vi "WaitForConnection.vi"(8 "error in (no error)":errorcluster, 11 "TcpServer in":refnum<class "TcpServer.lvclass">) -> (0 "error out":errorcluster, 3 "TcpServer out":refnum<class "TcpServer.lvclass">)   [LabVIEW 2022 SP3, in "TcpServer.lvlib" / "TcpServer.lvclass"]
uses:
  TcpServer.lvclass
  C:/Users/jakub/repos/gh/sw4sys/lv-tcp-server-sample/LoggingActor/Source/LoggingActor/LoggingActor/LoggingActor.lvclass
  C:/Program Files (x86)/National Instruments/LabVIEW 2022/vi.lib/ActorFramework/Actor/Actor.lvclass
  TcpServer.lvclass/TcpServer.ctl
  LoggingActor/Source/LoggingActor/LoggingActor/LoggingActor.lvclass/LoggingActor.ctl
  Connection/Connection/Connection.lvclass
  TcpSocket/Source/TcpSocket/Connection/Connection.lvclass/Connection.ctl
  Connection/Connection Messages/Initialize Msg/Initialize Msg.lvclass/Initialize Msg.ctl
  <vilib>/ActorFramework/Message Enqueuer/Message Enqueuer.lvclass/Message Enqueuer.ctl
  <vilib>/ActorFramework/Actor/Actor.lvclass/Actor.ctl
  TcpSocket/Source/TcpSocket/Connection/Read Address.vi
  TcpSocket/Source/TcpSocket/Connection/Read Port.vi
  TcpSocket/Source/TcpSocket/Connection/Read Connection.vi
  TcpSocket/Source/TcpSocket/Connection/Read ReadMode.vi
  TcpSocket/Source/TcpSocket/Connection/Read ReadTimeout.vi
  TcpSocket/Source/TcpSocket/Connection/Read WriteTimeout.vi
  LoggingActor/Source/LoggingActor/LoggingActor/Read Logger.vi
  <vilib>/ActorFramework/Message Enqueuer/Enqueue.vi
  <vilib>/ActorFramework/Message Enqueuer/Init from Existing Queue.vi
  Connection/Connection Messages/Initialize Msg/Initialize Msg.lvclass
  C:/Program Files (x86)/National Instruments/LabVIEW 2022/vi.lib/ActorFramework/Message/Message.lvclass
  TcpServer Messages/WaitForConnection Msg/WaitForConnection Msg.lvclass
  <vilib>/ActorFramework/Message Priority Queue/Priority Enqueue.vi
  Logger/Source/Logger/Logger.lvclass
  <vilib>/ActorFramework/Message Enqueuer/Message Enqueuer.lvclass
  TcpSocket/Source/TcpSocket/TcpServer/TcpServer.lvclass
  <vilib>/ActorFramework/Actor/Actor.lvclass
  TcpSocket/Source/TcpSocket/Connection/Connection.lvclass
  C:/Users/jakub/repos/gh/sw4sys/lv-tcp-server-sample/TcpServerSample/Source/TcpServerSample/Connection/Connection/Connection.lvclass
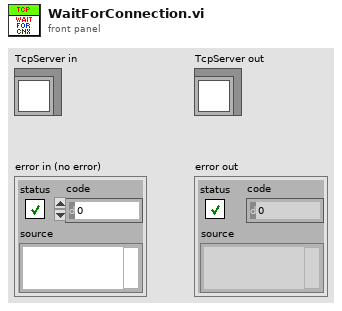
[diagram p1: front panel]
types:
  T1 = typedef "TcpServer.lvlib/TcpServer.lvclass/_ServerState.ctl" = enum16{"Idle", "Running"}
  T2 = map{u64, refnum<class "Message Enqueuer.lvclass">}
  T3 = enum16{"Standard", "Buffered", "CRLF", "Immediate"}
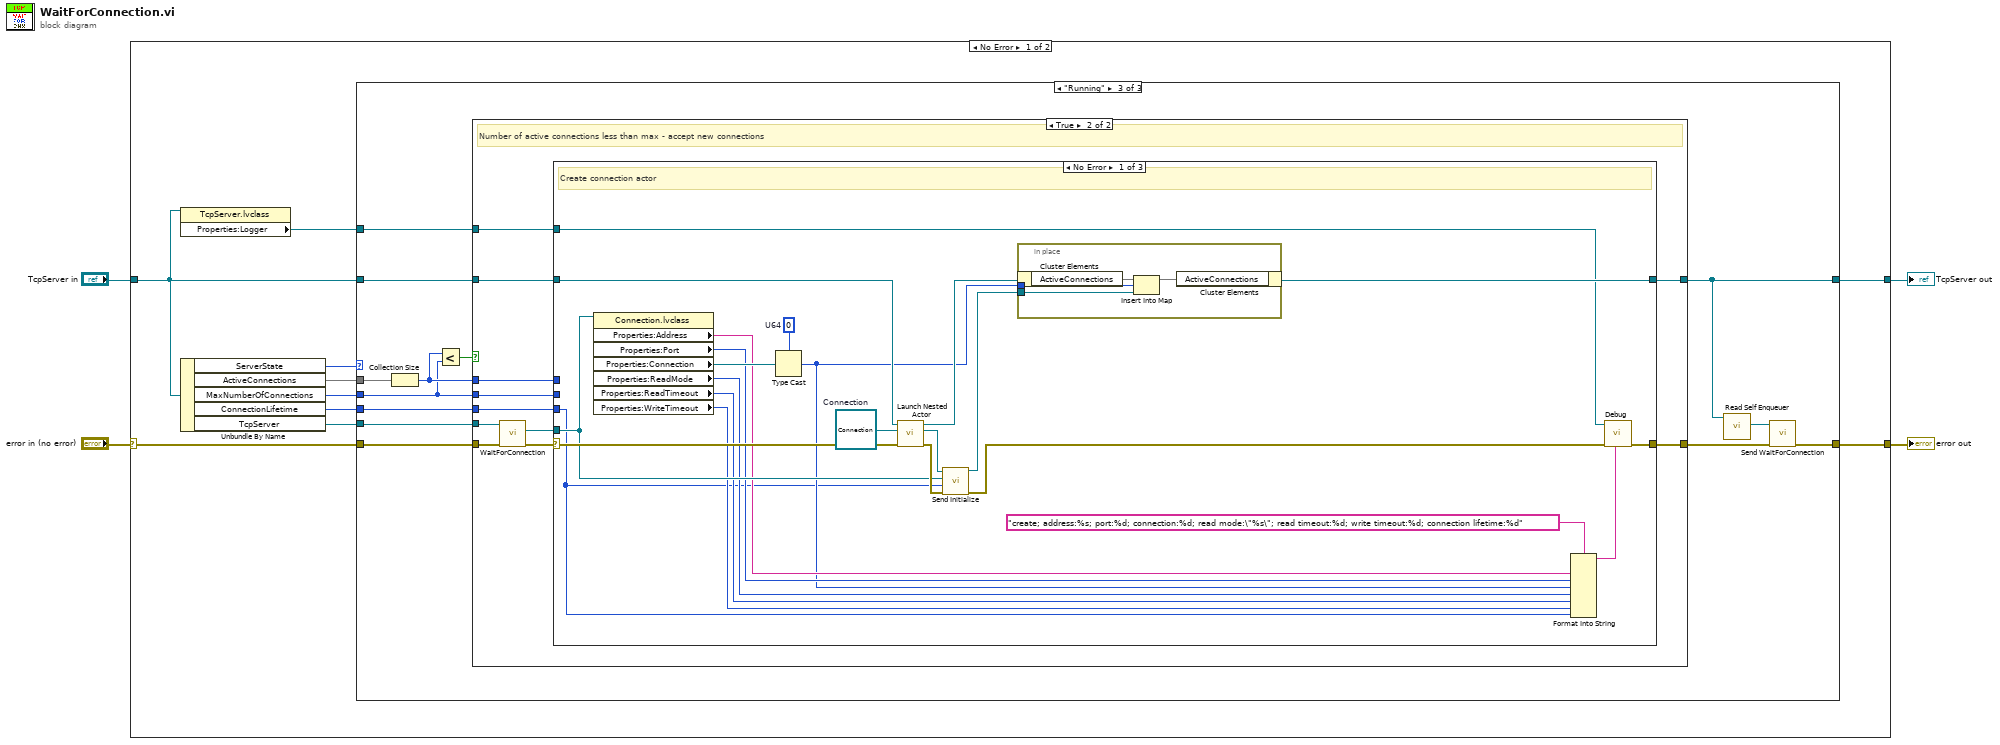
[diagram p0: block diagram]
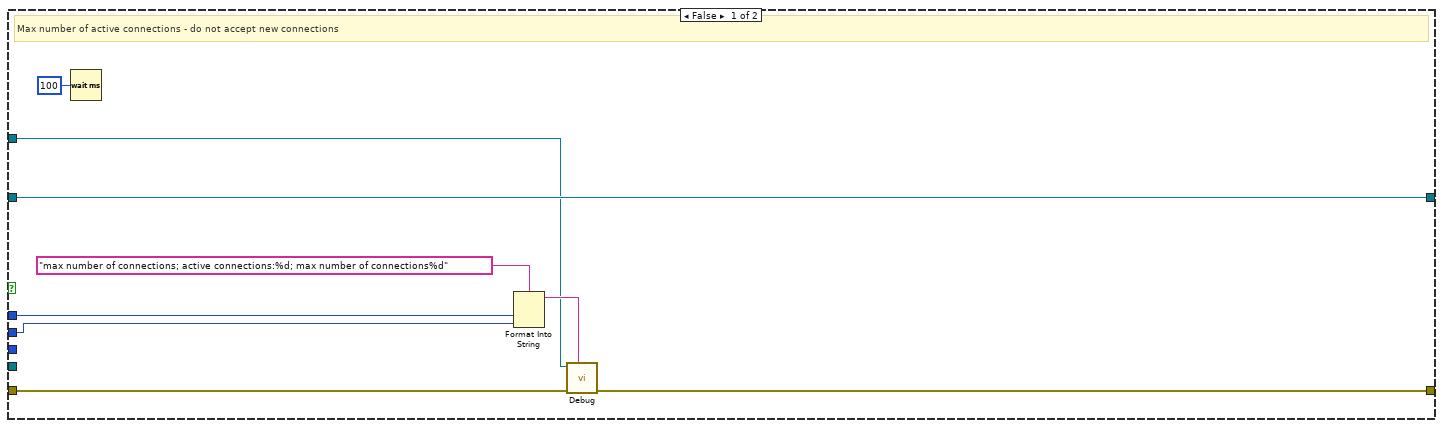
[diagram p4: hidden frame]
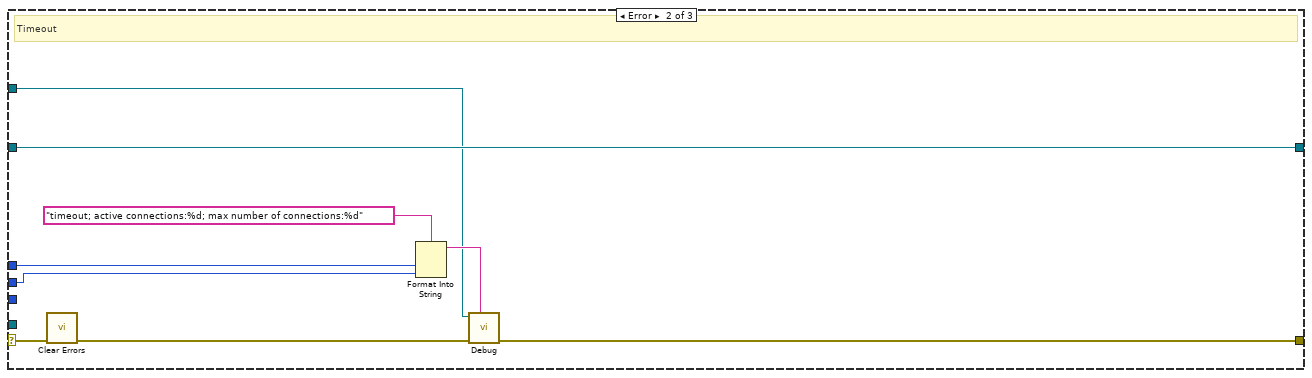
[diagram p5: hidden frame]
diagram:
  n1 = case shown="No Error" "error in (no error)" {
    selector: "error in (no error)" -> [w14 w91]
    tunnel: [w10 w91] -> w3
    tunnel: [w11 w90] -> w1
    tunnel: "TcpServer in" -> [w6 w90]
    frame No Error {
      n2 = property class="TcpServer.lvclass"(reference=w6) -> ("Properties:Logger"=w5:refnum<class "Logger.lvclass">)  [unwired: 1 in, 2 out]
      n3 = Unbundle By Name(w6) -> ("ServerState"=w7:T1, "ActiveConnections"=w9:T2, "MaxNumberOfConnections"=w8:i32, "ConnectionLifetime"=w12:i32, "TcpServer"=w13:refnum<class "TcpServer.lvclass">)
      n4 = case shown="\"Running\"" w7 {
        tunnel: w14 -> [w15 w17 w31]
        tunnel: w13 -> [_ _ w30]
        tunnel: w6 -> [w16 w18 w29]
        tunnel: w12 -> [_ _ w28]
        tunnel: [w16 w18 w27] -> w11
        tunnel: [w15 w17 w25] -> w10
        tunnel: w9 -> [_ _ w23]
        tunnel: w8 -> [_ _ w19]
        tunnel: w5 -> [_ _ w21]
        frame Default {
        }
        frame "Idle" {
        }
        frame "Running" {
          n5 = Collection Size(1:w23) -> (0:w20:i32)
          n6 = Less?(x=w20, y=w19) -> (x < y?=w22:bool)
          n7 = case shown="True" w22 {
            tunnel: w31 -> [w35 w51]
            tunnel: w30 -> [_ w48]
            tunnel: w29 -> [w40 w47]
            tunnel: w28 -> [_ w46]
            tunnel: [w40 w45] -> w27
            tunnel: [w36 w44] -> w26
            tunnel: w21 -> [w34 w43]
            tunnel: w20 -> [w33 w42]
            tunnel: w19 -> [w32 w41]
            frame False {
              # "Max number of active connections - do not accept new connections"
              n8 = Wait (ms)(milliseconds to wait=u32 100) -> ()  [unwired: 1 out]
              n9 = Format Into String(format string="max number of connections; active connections:%d; max number of connections%d", w33, w32) -> (resulting string=w37:string)  [unwired: 2 in, 1 out]
              n10 = call-dynamic "Debug.vi"("Message"=w37, "error in (no error)"=w35, "Logger in"=w34) -> ("error out"=w36:errorcluster)  [unwired: 5 in, 1 out]
            }
            frame True {
              # "Number of active connections less than max - accept new connections"
              n11 = call-dynamic "WaitForConnection.vi"("error in (no error)"=w51, "TcpServer in"=w48) -> ("error out"=w50:errorcluster, "Connection"=w49:refnum<class "Connection.lvclass">)  [unwired: 7 in, 1 out]
              n12 = case shown="No Error" w50 {
                selector: w50 -> [w74 w87 w89]
                tunnel: [w63 w84 w89] -> w44
                tunnel: w49 -> [w67 _ _]
                tunnel: w47 -> [w72 w86 w88]
                tunnel: [w62 w86 w88] -> w45
                tunnel: w46 -> [w54 _ _]
                tunnel: w43 -> [w52 w79 _]
                tunnel: w42 -> [_ w81 _]
                tunnel: w41 -> [_ w80 _]
                frame No Error {
                  w65 = u64 0  # U64
                  w73 = refnum<class "Connection.lvclass"> refnum  # Connection
                  # "Create connection actor"
                  n13 = property class="Connection.lvclass"(reference=w67) -> ("Properties:Address"=w60:string, "Properties:Port"=w59:u16, "Properties:Connection"=w66:refnum<k5>, "Properties:ReadMode"=w57:T3, "Properties:ReadTimeout"=w56:i32, "Properties:WriteTimeout"=w55:i32)  [unwired: 1 in, 2 out]
                  n14 = Type Cast(type=w65, x=w66) -> (*(type *) &x=w58:u64)
                  n15 = call <vilib>:"Launch Nested Actor.vi"("error in (no error)"=w74, "Nested Actor"=w73, "Caller Actor in"=w72) -> ("error out"=w70:errorcluster, "Nested Actor's Enqueuer"=w71:refnum<class "Message Enqueuer.lvclass">, "Caller Actor out"=w68:refnum<class "TcpServer.lvclass">)  [unwired: 6 in]
                  n16 = call "Send Initialize.vi"("error in (no error)"=w70, "Timeout [ms] (5000)"=w54, "Connection"=w67, "Message Enqueuer"=w71) -> ("error out"=w64:errorcluster, "Message Enqueuer out"=w69:refnum<class "Message Enqueuer.lvclass">)  [unwired: 6 in]
                  n17 = in-place {
                    in-place-border: w69 -> [w76]
                    in-place-border: w58 -> [w75]
                    n18 = in-place-cluster #1(w68) -> ("ActiveConnections"=w78:T2)
                    n19 = Insert Into Map(map in=w78, key=w75, value=w76) -> (map out=w77:T2)  [unwired: 2 out]
                    n20 = in-place-cluster #1("ActiveConnections"=w77) -> (w62:refnum<class "TcpServer.lvclass">)
                  }
                  n21 = Format Into String(format string="create; address:%s; port:%d; connection:%d; read mode:\"%s\"; read timeout:%d; write timeout:%d; connection lifetime:%d", w60, w59, w58, w57, w56, w55, w54) -> (resulting string=w53:string)  [unwired: 2 in, 1 out]
                  n22 = call-dynamic "Debug.vi"("Message"=w53, "error in (no error)"=w64, "Logger in"=w52) -> ("error out"=w63:errorcluster)  [unwired: 5 in, 1 out]
                }
                frame Error {
                  # "Timeout"
                  n23 = call <vilib>:"Clear Errors.vi"("error in (no error)"=w87) -> ("error out"=w85:errorcluster)  [unwired: 5 in, 1 out]
                  n24 = Format Into String(format string="timeout; active connections:%d; max number of connections:%d", w81, w80) -> (resulting string=w82:string)  [unwired: 2 in, 1 out]
                  n25 = call-dynamic "Debug.vi"("Message"=w82, "error in (no error)"=w85, "Logger in"=w79) -> ("error out"=w84:errorcluster)  [unwired: 5 in, 1 out]
                }
                frame Default {
                  # "Error"
                }
              }
            }
          }
          n26 = call <vilib>:"Read Self Enqueuer.vi"("Actor"=w27) -> ("Self Enqueuer"=w24:refnum<class "Message Enqueuer.lvclass">)  [unwired: 10 in]
          n27 = call "Send WaitForConnection.vi"("error in (no error)"=w26, "Message Enqueuer"=w24) -> ("error out"=w25:errorcluster)  [unwired: 8 in, 1 out]
        }
      }
    }
    frame Error {
    }
  }
  "error out" <- w3
  "TcpServer out" <- w1
